vi "Kicker.vi"(5 "IA State Input":T1={"our_robots"=[], "enemy_robots"=[], "balls"=[], "geometry"={"line_width"=0, "field_length"=0, "field_width"=0, "boundary_width"=0, "referee_width"=0, "goal_width"=0, "goal_depth"=0, "goal_wall_width"=0, "center_circle_radius"=0, "defense_radius"=0, "defense_stretch"=0, "free_kick_from_defense_dist"=0, "penalty_spot_from_field_line_dist"=0, "penalty_line_from_spot_dist"=0}, "IA Judge"={"stage"="", "command"="", "our_goalie_id"=0.0, "enemy_goalie_id"=0.0, "command\nenum"=enum."Halt", "Time"=enum."Azul"}, "Received Timestamp"=timestamp(0 s since 1904-01-01), "Events"={"Touch"=FALSE, "Ball out"=FALSE, "id touch"=0.0, "Ball out of \nVision"=FALSE, "Ball inside \nGoalie area"=FALSE, "Robot not responding"=FALSE, "Robots responding status"=[1.0, 1.0, 1.0, 1.0, 1.0, 1.0]}}, 7 "Dribble":bool, 8 "Ball velocity":dbl[](array[numeric]), 9 "Vel_kick":dbl=5.0 format="%#_13g", 10 "Kick?":bool, 11 "Robot in":T2={"id"=5, "function"=enum."Attacker", "x"=-983.1382446289062, "y"=-3000.010498046875, "orientation"=-1.5516623258590698, "v_tangent"=0.0, "v_normal"=0.0, "v_ang"=0.0, "kick_x"=0.0, "kick_z"=0.0, "dribble"=FALSE, "Timestamp"=timestamp(2082759045.994995 s since 1904-01-01), "dest_x"=0.0, "dest_y"=0.0, "dest_orientation"=0.0, "estimatives"={"est_v_tangent"=0.0, "est_v_normal"=0.0, "est_vx"=0.0, "est_vy"=0.0}, "dest_x_kick"=0.0, "dest_y_kick"=0.0, "Gap Coord"=[]}) -> (2 "output cluster":T2)   [LabVIEW 2016]
uses:
  Core/AI Robot.ctl
  Functions Enum.ctl
  Core/AI Input.ctl
  Core/AI Ball.ctl
  Core/Field Size.ctl
  Core/AI Judge.ctl
  Command Enum.ctl
panel:
  in  "gravar":bool=TRUE
  in  "Vel min to write":dbl format="%#_13g"
  in  "file path (use dialog)":path=path "C:/Users/Robótica/git/SSLView/Farias.csv"
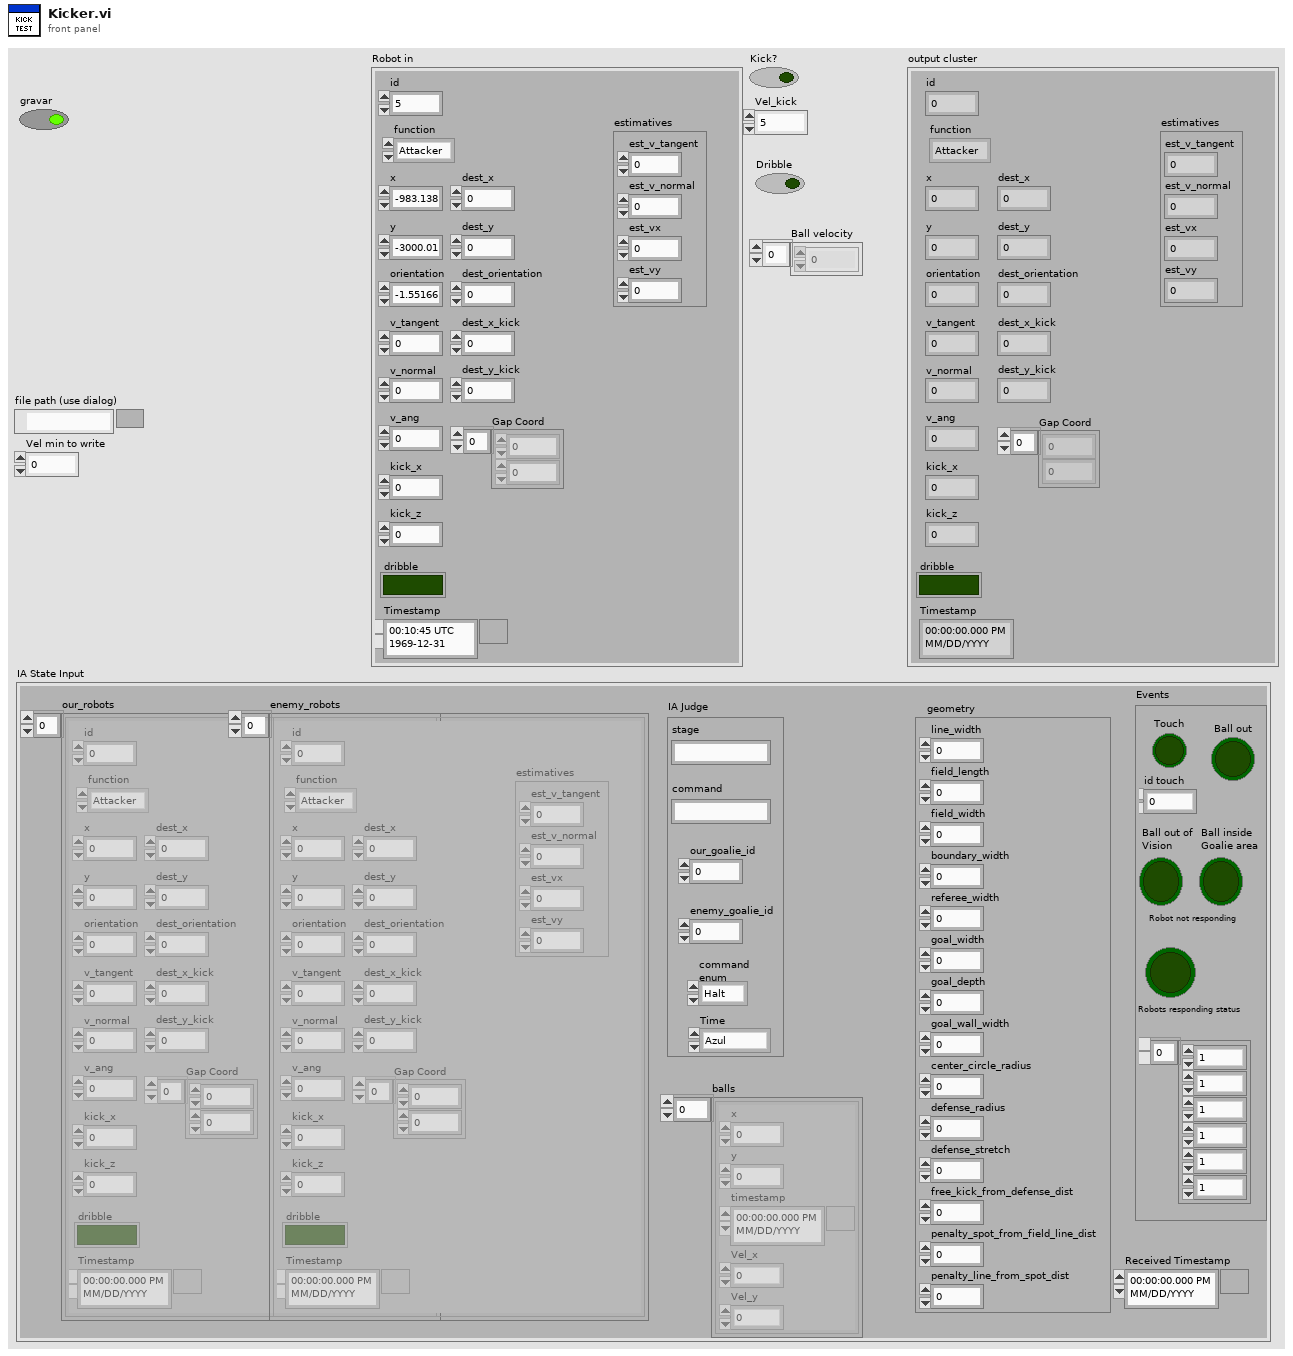
[diagram p1: front panel]
types:
  T1 = typedef "AI Input.ctl" = cluster{"our_robots":T2[], "enemy_robots":T2[], "balls":T4[], "geometry":T5, "IA Judge":T6, "Received Timestamp":timestamp, "Events":cluster{"Touch":bool, "Ball out":bool, "id touch":dbl, "Ball out of \nVision":bool, "Ball inside \nGoalie area":bool, "Robot not responding":bool, "Robots responding status":dbl[]}}
  T2 = typedef "AI Robot.ctl" = cluster{"id":u32, "function":T3, "x":dbl, "y":dbl, "orientation":dbl, "v_tangent":dbl, "v_normal":dbl, "v_ang":dbl, "kick_x":dbl, "kick_z":dbl, "dribble":bool, "Timestamp":timestamp, "dest_x":dbl, "dest_y":dbl, "dest_orientation":dbl, "estimatives":cluster{"est_v_tangent":dbl, "est_v_normal":dbl, "est_vx":dbl, "est_vy":dbl}, "dest_x_kick":dbl, "dest_y_kick":dbl, "Gap Coord":dbl[]}
  T3 = typedef "Functions Enum.ctl" = enum16{"Attacker", "Goalie", "Defender", "Striker", "Goto 0", "Dummy", "Kicker", "ZigZag"}
  T4 = typedef "AI Ball.ctl" = cluster{"x":dbl, "y":dbl, "timestamp":timestamp, "Vel_x":dbl, "Vel_y":dbl}
  T5 = typedef "Field Size.ctl" = cluster{"line_width":u32, "field_length":u32, "field_width":u32, "boundary_width":u32, "referee_width":u32, "goal_width":u32, "goal_depth":u32, "goal_wall_width":u32, "center_circle_radius":u32, "defense_radius":u32, "defense_stretch":u32, "free_kick_from_defense_dist":u32, "penalty_spot_from_field_line_dist":u32, "penalty_line_from_spot_dist":u32}
  T6 = typedef "AI Judge.ctl" = cluster{"stage":string, "command":string, "our_goalie_id":dbl, "enemy_goalie_id":dbl, "command\nenum":T7, "Time":enum16{"Azul", "Amarelo"}}
  T7 = typedef "Command Enum.ctl" = enum16{"Halt", "Stop", "Force Start", "PKA Normal Start", "Prepare Kickoff Ally", "PKE Normal Start", "Prepare Kickoff Enemy", "Prepare Penalty Ally", "PPA Normal Start", "Prepare Penalty Enemy", "PPE Normal Start", "Direct Free Enemy", "Direct Free Ally", "Indirect Free Enemy", "Indirect Free Ally", "Timeout Enemy", "Timeout Ally", "Goal Enemy", "Goal Ally", "Ball Placement Enemy", "Ball Placement Ally", "None"}
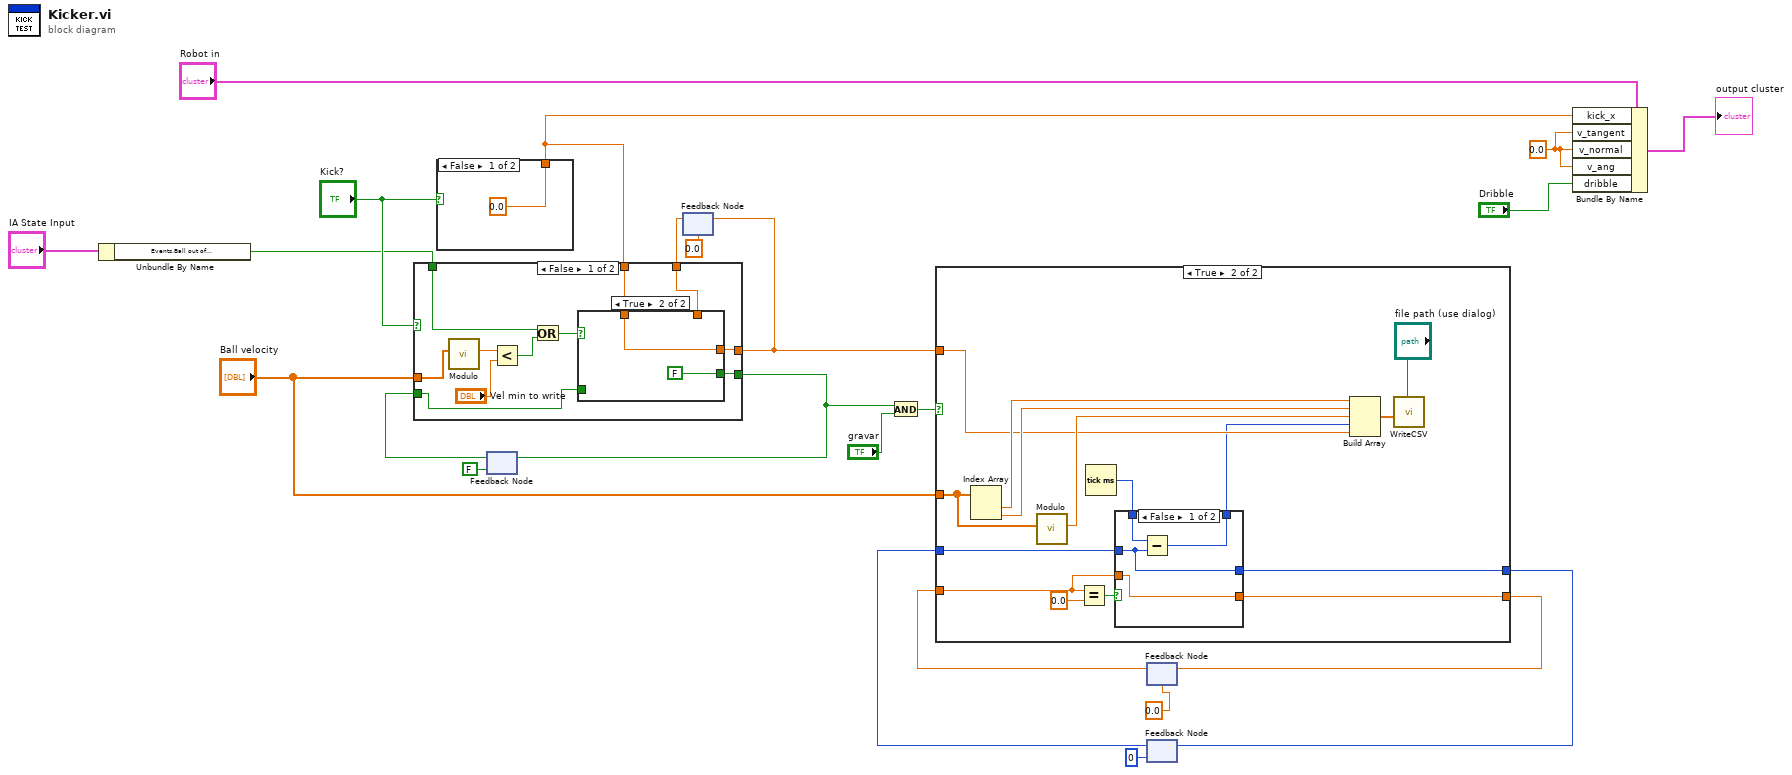
[diagram p0: block diagram]
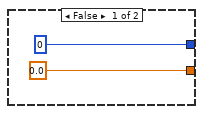
[diagram p2: hidden frame]
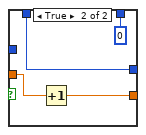
[diagram p3: hidden frame]
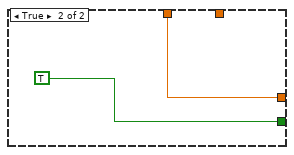
[diagram p5: hidden frame]
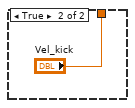
[diagram p6: hidden frame]
diagram:
  w21 = 0.0 ("v_normal")
  n1 = Unbundle By Name("IA State Input") -> ("Events.Ball out of \nVision"=w16:bool)
  n2 = case shown="False" "Kick?" {
    tunnel: [0.0 "Vel_kick"] -> w13
    frame False {
    }
    frame True {
    }
  }
  n3 = feedback #1(FALSE) -> (w18:bool)
  n4 = feedback #2(0.0 ("Vel_kick")) -> (w12:dbl)
  n5 = case shown="False" "Kick?" {
    tunnel: [w30 TRUE] -> w1
    tunnel: w18 -> [w29 _]
    tunnel: "Ball velocity" -> [w35 _]
    tunnel: w16 -> [w31 _]
    tunnel: w13 -> [w27 w41]
    tunnel: [w28 w41] -> w8
    tunnel: w12 -> [w26 _]
    frame False {
      n6 = call "Modulo.vi"("2D vector"=w35) -> ("Modulo"=w36:dbl)  [unwired: 10 in]
      n7 = Less?(x=w36, y="Vel min to write") -> (x < y?=w32:bool)
      n8 = Or(x=w31, y=w32) -> (x .or. y?=w33:bool)
      n9 = case shown="True" w33 {
        tunnel: [w38 FALSE] -> w30
        tunnel: w29 -> [w38 _]
        tunnel: [w37 w39] -> w28
        tunnel: w27 -> [_ w39]
        tunnel: w26 -> [w37 _]
        frame False {
        }
        frame True {
        }
      }
    }
    frame True {
    }
  }
  n10 = feedback-in #1(w1) -> ()
  n11 = feedback-in #2(w8) -> ()
  n12 = And(x=w1, y="gravar") -> (x .and. y?=w10:bool)
  n13 = feedback #3(0.0) -> (w6:dbl)
  n14 = feedback #4(u32 0 ("millisecond timer value")) -> (w3:u32)
  n15 = case shown="True" w10 {
    tunnel: "Ball velocity" -> [_ w55]
    tunnel: w8 -> [_ w53]
    tunnel: [0.0 w51] -> w7
    tunnel: w6 -> [_ w48]
    tunnel: [u32 0 ("millisecond timer value") w46] -> w4
    tunnel: w3 -> [_ w47]
    frame False {
    }
    frame True {
      n16 = Index Array(array=w55) -> (element #1=w59:dbl, element #2=w56:dbl)  [unwired: 2 in]
      n17 = call "Modulo.vi"("2D vector"=w55) -> ("Modulo"=w54:dbl)  [unwired: 10 in]
      n18 = Equal?(x=w48, y=0.0) -> (x = y?=w50:bool)
      n19 = Tick Count (ms)() -> (millisecond timer value=w52:u32)
      n20 = case shown="False" w50 {
        tunnel: w52 -> [w63 w65]
        tunnel: [w62 w67] -> w51
        tunnel: w48 -> [w62 w66]
        tunnel: [w61 w65] -> w46
        tunnel: w47 -> [w61 _]
        tunnel: [w60 u32 0] -> w45
        frame False {
          n21 = Subtract(x=w63, y=w61) -> (x-y=w60:u32)
        }
        frame True {
          n22 = Increment(x=w66) -> (x+1=w67:dbl)
        }
      }
      n23 = Build Array(w59, w56, w54, w45, w53) -> (w58:dbl[])
      n24 = call "WriteCSV.vi"("array"=w58, "file path (use dialog)"="file path (use dialog)") -> ()  [unwired: 10 in]
    }
  }
  n25 = feedback-in #3(w7) -> ()
  n26 = feedback-in #4(w4) -> ()
  n27 = Bundle By Name(cluster="Robot in", "kick_x"=w13, "v_tangent"=w21, "v_normal"=w21, "v_ang"=w21, "dribble"="Dribble") -> (→"output cluster":T2)
